vi "Get Messages for Connection Lists.vi"(6 "Message Type":enum16{"Connect", "Disconnect"}(ring), 8 "error in (no error)":errorcluster, 9 "Compiled Connection Buffer":T1[](array[typedef]), 10 "Communication Configuration":T3, 11 "Connection Lists for each Module":cluster{"Indices":i32[]}[](array[cluster])) -> (0 "error out":errorcluster, 3 "Messages":T2[](array[typedef]))   [LabVIEW 2017, in "Routing and Faulting Engine.lvlib"]
uses:
  Routing and Faulting Engine.lvlib
  Shared/Communication Configuration.ctl
  Producer Message.ctl
  Includes/CDMessaging.lvlibp/Message/Abstract Message/Abstract Message.lvclass
  Shared/Compiled Connection.ctl
  Includes/CDMessaging.lvlibp/Switch/Switch Connect Message/Switch Connect Message.lvclass
  C:/Users/nitest/Documents/ni-official/niveristand-routing-and-faulting-custom-device/Includes/CDMessaging.lvlibp/Message/Abstract Request Message/Abstract Request Message.lvclass
  Includes/CDMessaging.lvlibp/Switch/Switch Disconnect Message/Switch Disconnect Message.lvclass
  Includes/CDMessaging.lvlibp/Message/Abstract Request Message/Abstract Request Message.lvclass
  C:/Users/nitest/Documents/ni-official/niveristand-routing-and-faulting-custom-device/Includes/CDMessaging.lvlibp/Message/Abstract Message/Abstract Message.lvclass
  Shared/Routing and Faulting Shared.lvlib
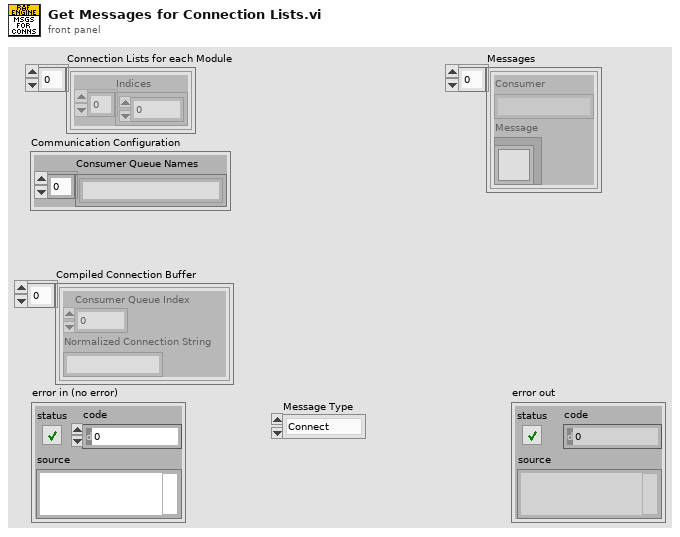
[diagram p1: front panel]
types:
  T1 = typedef "Routing and Faulting Shared.lvlib/Compiled Connection.ctl" = cluster{"Consumer Queue Index":i32, "Normalized Connection String":string}
  T2 = typedef "Routing and Faulting Engine.lvlib/Producer Message.ctl" = cluster{"Consumer":string, "Message":refnum<class "Abstract Message.lvclass">}
  T3 = typedef "Routing and Faulting Shared.lvlib/Communication Configuration.ctl" = cluster{"Consumer Queue Names":string[]}
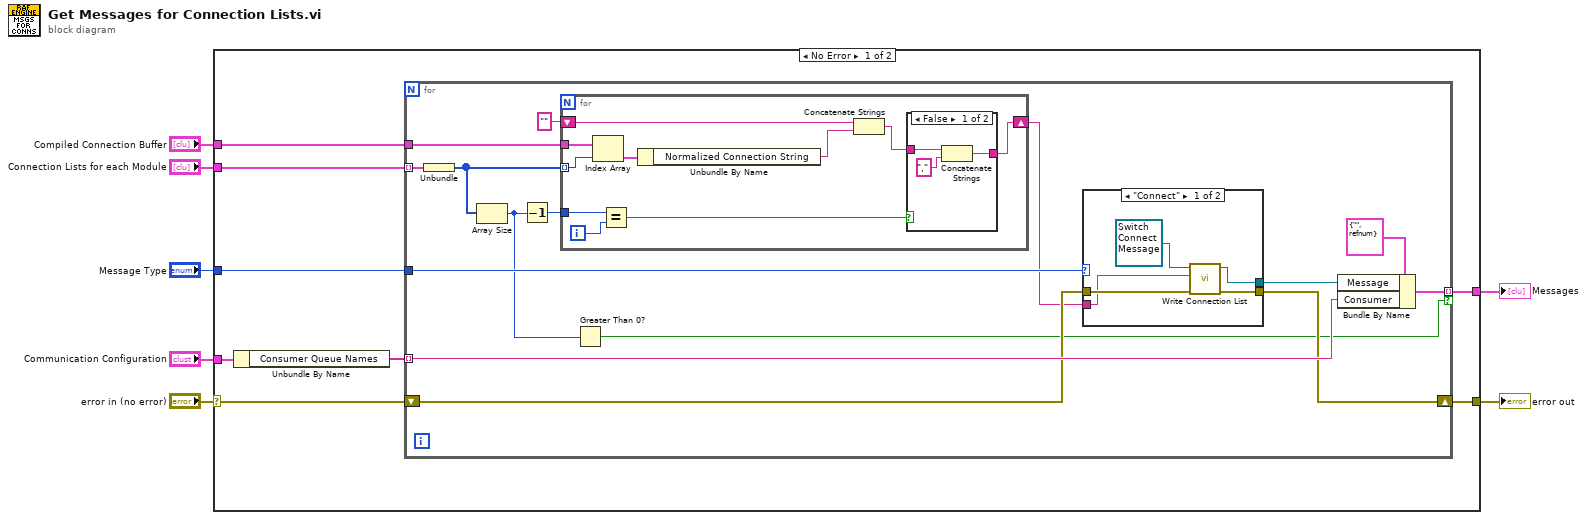
[diagram p0: block diagram]
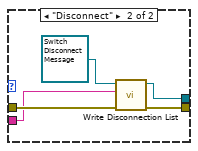
[diagram p3: hidden frame]
diagram:
  n1 = case shown="No Error" "error in (no error)" {
    selector: "error in (no error)" -> [w11 w55]
    tunnel: "Communication Configuration" -> [w15 _]
    tunnel: "Connection Lists for each Module" -> [w13 _]
    tunnel: [w12 _] -> w6
    tunnel: [w10 w55] -> w4
    tunnel: "Message Type" -> [w9 _]
    tunnel: "Compiled Connection Buffer" -> [w8 _]
    frame No Error {
      n2 = Unbundle By Name(w15) -> ("Consumer Queue Names"=w14:string[])
      n3 = for {
        tunnel: w13 -> [w30] mode=indexing
        tunnel: w14 -> [w27] mode=indexing
        tunnel: [w26] -> w12 mode=indexing if=w19
        shift-right: [w24] -> w10
        shift-left: w11 -> [w25]
        tunnel: w9 -> [w23]
        tunnel: w8 -> [w16]
        n4 = Unbundle(w30) -> ("Indices"=w20:i32[])
        n5 = Array Size(array=w20) -> (size(s)=w18:i32)
        n6 = Decrement(x=w18) -> (x-1=w17:i32)
        n7 = for {
          tunnel: w20 -> [w35] mode=indexing
          shift-right: [w37] -> w22
          shift-left: "" -> [w34]
          tunnel: w17 -> [w40]
          tunnel: w16 -> [w36]
          i -> [w39]
          n8 = Index Array(array=w36, index=w35) -> (element=w32:T1)
          n9 = Equal?(x=w40, y=w39) -> (x = y?=w38:bool)
          n10 = Unbundle By Name(w32) -> ("Normalized Connection String"=w31:string)
          n11 = Concatenate Strings(w34, w31) -> (w33:string)
          n12 = case shown="False" w38 {
            tunnel: w33 -> [w43 w44]
            tunnel: [w42 w44] -> w37
            frame False {
              n13 = Concatenate Strings(w43, "," ("string")) -> (w42:string)
            }
            frame True {
            }
          }
        }
        n14 = Greater Than 0?(x=w18) -> (x > 0?=w19:bool)
        n15 = case shown="\"Connect\"" w23 {
          tunnel: w22 -> [w46 w51]
          tunnel: [w45 w50] -> w28
          tunnel: w25 -> [w48 w53]
          tunnel: [w47 w54] -> w24
          frame "Connect" {
            n16 = call-dynamic "Write Connection List.vi"("error in (no error)"=w48, "Connection List"=w46, "Switch Connect Message in"=refnum<class "Switch Connect Message.lvclass"> refnum ("CDMessaging.lvlibp:Switch Connect Message.lvclass")) -> ("error out"=w47:errorcluster, "Switch Connect Message out"=w45:refnum<class "Switch Connect Message.lvclass">)  [unwired: 7 in]
          }
          frame "Disconnect" {
            n17 = call-dynamic "Write Disconnection List.vi"("error in (no error)"=w53, "Disconnection List"=w51, "Switch Disconnect Message in"=refnum<class "Switch Disconnect Message.lvclass"> refnum ("CDMessaging.lvlibp:Switch Disconnect Message.lvclass")) -> ("error out"=w54:errorcluster, "Switch Disconnect Message out"=w50:refnum<class "Switch Disconnect Message.lvclass">)  [unwired: 7 in]
          }
        }
        n18 = Bundle By Name(cluster=T2 {"Consumer"="", "Message"=refnum} ("Producer Message"), "Message"=w28, "Consumer"=w27) -> (w26:T2)
      }
    }
    frame Error {
    }
  }
  "Messages" <- w6
  "error out" <- w4
